vi "Check Parent Folder Selection.vi"(0 "Tree reference in":refnum<vi>, 5 "Child Tag":string, 11 "error in":errorcluster) -> (4 "Tree reference out":refnum<vi>, 15 "error out":errorcluster)   [LabVIEW 2021, in "Migrator.lvlib"]
uses:
  Migrator.lvlib
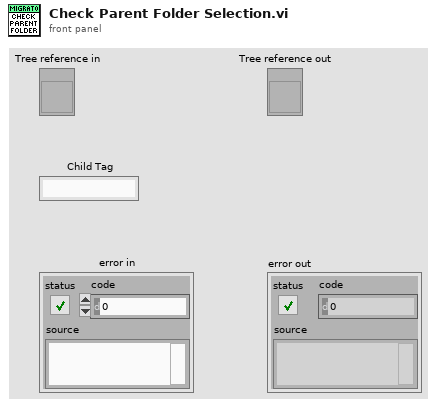
[diagram p1: front panel]
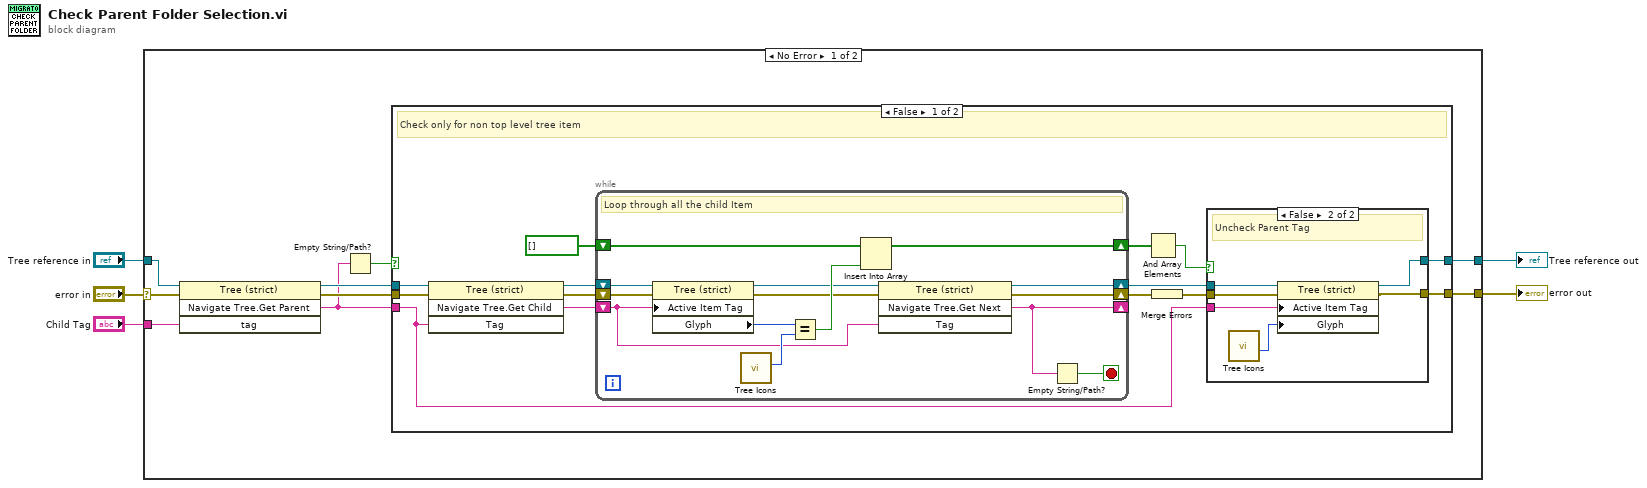
[diagram p0: block diagram]
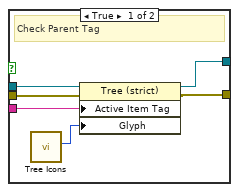
[diagram p2: hidden frame]
diagram:
  n1 = case shown="No Error" "error in" {
    selector: "error in" -> [w13 w58]
    tunnel: "Child Tag" -> [w14 _]
    tunnel: "Tree reference in" -> [w10 w57]
    tunnel: [w7 w58] -> w2
    tunnel: [w6 w57] -> w1
    frame No Error {
      n2 = invoke class="Tree (strict)" method="Navigate Tree.Get Parent"(reference=w10, error in=w13, "tag"=w14) -> (reference out=w12:refnum<vi>, error out=w11:errorcluster, "Navigate Tree:Get Parent"=w8:string)  [unwired: 1 in, 1 out]
      n3 = Empty String/Path?(string/path=w8) -> (empty?=w9:bool)
      n4 = case shown="False" w9 {
        tunnel: w12 -> [w28 w55]
        tunnel: w8 -> [w19 _]
        tunnel: w11 -> [w27 w56]
        tunnel: [w18 w56] -> w7
        tunnel: [w15 w55] -> w6
        frame False {
          # "Check only for non top level tree item"
          n5 = invoke class="Tree (strict)" method="Navigate Tree.Get Child"(reference=w28, error in=w27, "Tag"=w19) -> (reference out=w24:refnum<vi>, error out=w25:errorcluster, "Navigate Tree:Get Child"=w26:string)  [unwired: 1 in, 1 out]
          n6 = while {
            shift-right: [w30] -> _
            shift-left: w26 -> [w32]
            shift-right: [w36] -> w16
            shift-left: w24 -> [w41]
            shift-right: [w31] -> w21
            shift-left: bool[] [] -> [w38]
            shift-right: [w34] -> w22
            shift-left: w25 -> [w42]
            stop <- w29 stop-if-true
            # "Loop through all the child Item"
            n7 = property class="Tree (strict)"(reference=w41, error in=w42, "Active Item Tag"=w32) -> (reference out=w33:refnum<vi>, error out=w35:errorcluster, "Glyph"=w39:i32)
            n8 = call "Tree Icons.vi"() -> ("Selected"=w40:i32)  [unwired: 6 in, 1 out]
            n9 = Equal?(x=w39, y=w40) -> (x = y?=w37:bool)
            n10 = Insert Into Array(array=w38, new element=w37) -> (w31:bool[])  [unwired: 1 in]
            n11 = invoke class="Tree (strict)" method="Navigate Tree.Get Next"(reference=w33, error in=w35, "Tag"=w32) -> (reference out=w36:refnum<vi>, error out=w34:errorcluster, "Navigate Tree:Get Next Item"=w30:string)  [unwired: 1 in, 1 out]
            n12 = Empty String/Path?(string/path=w30) -> (empty?=w29:bool)
          }
          n13 = And Array Elements(Boolean array=w21) -> (logical AND=w17:bool)
          n14 = Merge Errors(w22) -> (w20:errorcluster)
          n15 = case shown="False" w17 {
            tunnel: w20 -> [w48 w54]
            tunnel: w19 -> [w47 w53]
            tunnel: [w46 w52] -> w18
            tunnel: w16 -> [w44 w50]
            tunnel: [w43 w49] -> w15
            frame True {
              # "Check Parent Tag"
              n16 = call "Tree Icons.vi"() -> ("Selected"=w45:i32)  [unwired: 6 in, 1 out]
              n17 = property class="Tree (strict)"(reference=w44, error in=w48, "Active Item Tag"=w47, "Glyph"=w45) -> (reference out=w43:refnum<vi>, error out=w46:errorcluster)
            }
            frame False {
              # "Uncheck Parent Tag"
              n18 = call "Tree Icons.vi"() -> ("Not Selected"=w51:i32)  [unwired: 6 in, 1 out]
              n19 = property class="Tree (strict)"(reference=w50, error in=w54, "Active Item Tag"=w53, "Glyph"=w51) -> (reference out=w49:refnum<vi>, error out=w52:errorcluster)
            }
          }
        }
        frame True {
          # "Skip if top level tree item"
        }
      }
    }
    frame Error {
    }
  }
  "error out" <- w2
  "Tree reference out" <- w1
